vi "Main.vi"(11 "Module Admin":refnum<class "Delacor_lib_QMH_Module Admin.lvclass">) -> ()   [LabVIEW 2020, in "horiba.lvlib" / "DeviceManager.lvlib"]
doc: "This template is based off of the Queued Message Handler design pattern and the Queued Message Handler project template that ships with LabVIEW.\n\nThe main difference is that the queue is private to this module and communication between modules is performed via Broadcast and Request events.\n\nRequest events are wrapped in public API methods and are handled in the Event Handling Loop (EHL) of this VI. Any module can register for Broadcast events sent by this module. The EHL generates messages based on user interface actions.\n\nThe Message Handling Loop (MHL) processes messages generated by the EHL, or by other messages. The messages are string values, so new messages can be added easily to the Message Cases case structure in the MHL. Each message cluster can also provide an optional value for Message Data, which is a variant that can be converted to whatever message-specific data is required.\n_____\nBased on DQMH Project Template 7.0.0.1280."
uses:
  DeviceManager.lvlib
  <vilib>/Delacor/Delacor QMH/Libraries/Message Queue_class/Delacor_lib_QMH_Message Queue.lvclass
  Module Data--cluster.ctl
  <vilib>/Utility/miscctls.llb/LVPointTypeDef.ctl
  <vilib>/Delacor/Delacor QMH/Libraries/Message Queue_class/Delacor_lib_QMH_Enqueue Message (Single).vi
  Stop Argument--cluster.ctl
  <vilib>/Delacor/Delacor QMH/Libraries/Module Admin_class/Delacor_lib_QMH_Module Admin.lvclass
  OpenWebSocketCommunication (Reply Payload)--cluster.ctl
  ICLcommuncationData.ctl
  <vilib>/GPower/Error/GPError.lvlib
  Communicator/Communicator.lvclass
  SendJSONandAskForReply (Reply Payload)--cluster.ctl
  Mono/Monochromator.lvclass
  CCD/CCD.lvclass
  SCD/SCD.lvclass
  DiscoverDevices (Reply Payload)--cluster.ctl
  DevicesList (Reply Payload)--cluster.ctl
  18cac8b0-4f25-4128-b3b0-f125cc614320.vi
  3b3cd88e-03c4-4dd7-b5f0-8a6c9de4e459.vi
  89821459-91c3-422b-9ff8-53e1432d37b0.vi
  <vilib>/Hampel Software Engineering/HSE Logger/hse-logger.lvlib
panel:
  out "error out":errorcluster
  out "Status":string
  in  "Simulate MHL Error":bool
  in  "Simulate EHL Error":bool
  # "Device Manager"
  # "This DQMH module starts the Instrument Control Layer (ICL)\nand proved means to send messages to the ICL via websocket\ncommunication."
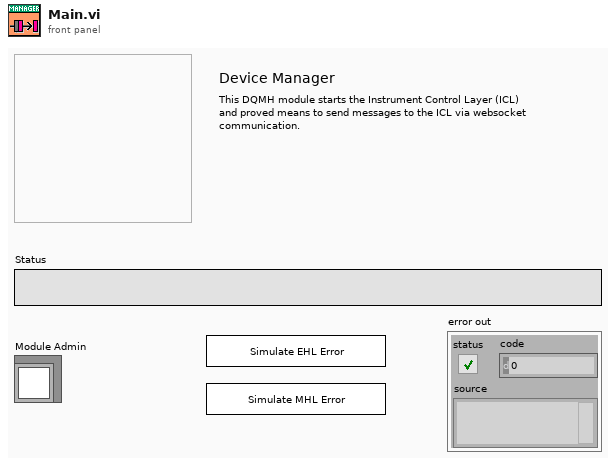
[diagram p1: front panel]
types:
  T1 = typedef "horiba.lvlib/DeviceManager.lvlib/Request Events--cluster.ctl" = cluster{"Stop Module":refnum<user-event>, "Show Panel":refnum<user-event>, "Hide Panel":refnum<user-event>, "Get Module Execution Status":refnum<user-event>, "Show Diagram":refnum<user-event>, "StartICL":refnum<user-event>, "OpenWebSocketCommunication":refnum<user-event>, "Private":cluster{"ICLstartNotification":refnum<user-event>}, "ICLshutdown":refnum<user-event>, "SendJSONandAskForReply":refnum<user-event>, "DiscoverDevices":refnum<user-event>, "DevicesList":refnum<user-event>}
  T2 = typedef "horiba.lvlib/DeviceManager.lvlib/ICLcommuncationData.ctl" = cluster{"Status":string, "ICL.exe started":bool, "Communicator":refnum<class "Communicator.lvclass">}
  T3 = typedef "horiba.lvlib/DeviceManager.lvlib/Module Data--cluster.ctl" = cluster{"Status":string}
  T4 = enum32{"invalid lock state", "Not Locked", "Locked (No Password)", "Password-protected"}
  T5 = typedef "horiba.lvlib/DeviceManager.lvlib/Stop Argument--cluster.ctl" = cluster{"Origin":string, "Exit via Stop Module Req?":bool, "Wait for Module to stop?":bool}
  T6 = typedef "LVPointTypeDef.ctl" = cluster{"Horizontal":i16, "Vertical":i16}
  T7 = enum32{"Invalid", "Standard", "Closed", "Hidden", "Minimized", "Maximized"}
  T8 = typedef "horiba.lvlib/DeviceManager.lvlib/OpenWebSocketCommunication (Reply Payload)--cluster.ctl" = cluster{"Return Headers":variant, "error":errorcluster}
  T9 = typedef "horiba.lvlib/DeviceManager.lvlib/SendJSONandAskForReply (Reply Payload)--cluster.ctl" = cluster{"JSON reply":string, "error":errorcluster}
  T10 = typedef "horiba.lvlib/DeviceManager.lvlib/DiscoverDevices (Reply Payload)--cluster.ctl" = cluster{"Monos":refnum<class "Monochromator.lvclass">[], "CCDs":refnum<class "CCD.lvclass">[], "SCDs":refnum<class "SCD.lvclass">[], "error":errorcluster}
  T11 = typedef "horiba.lvlib/DeviceManager.lvlib/DevicesList (Reply Payload)--cluster.ctl" = cluster{"monochromator results":string, "CCD-results":string, "SCD-results":string, "error":errorcluster}
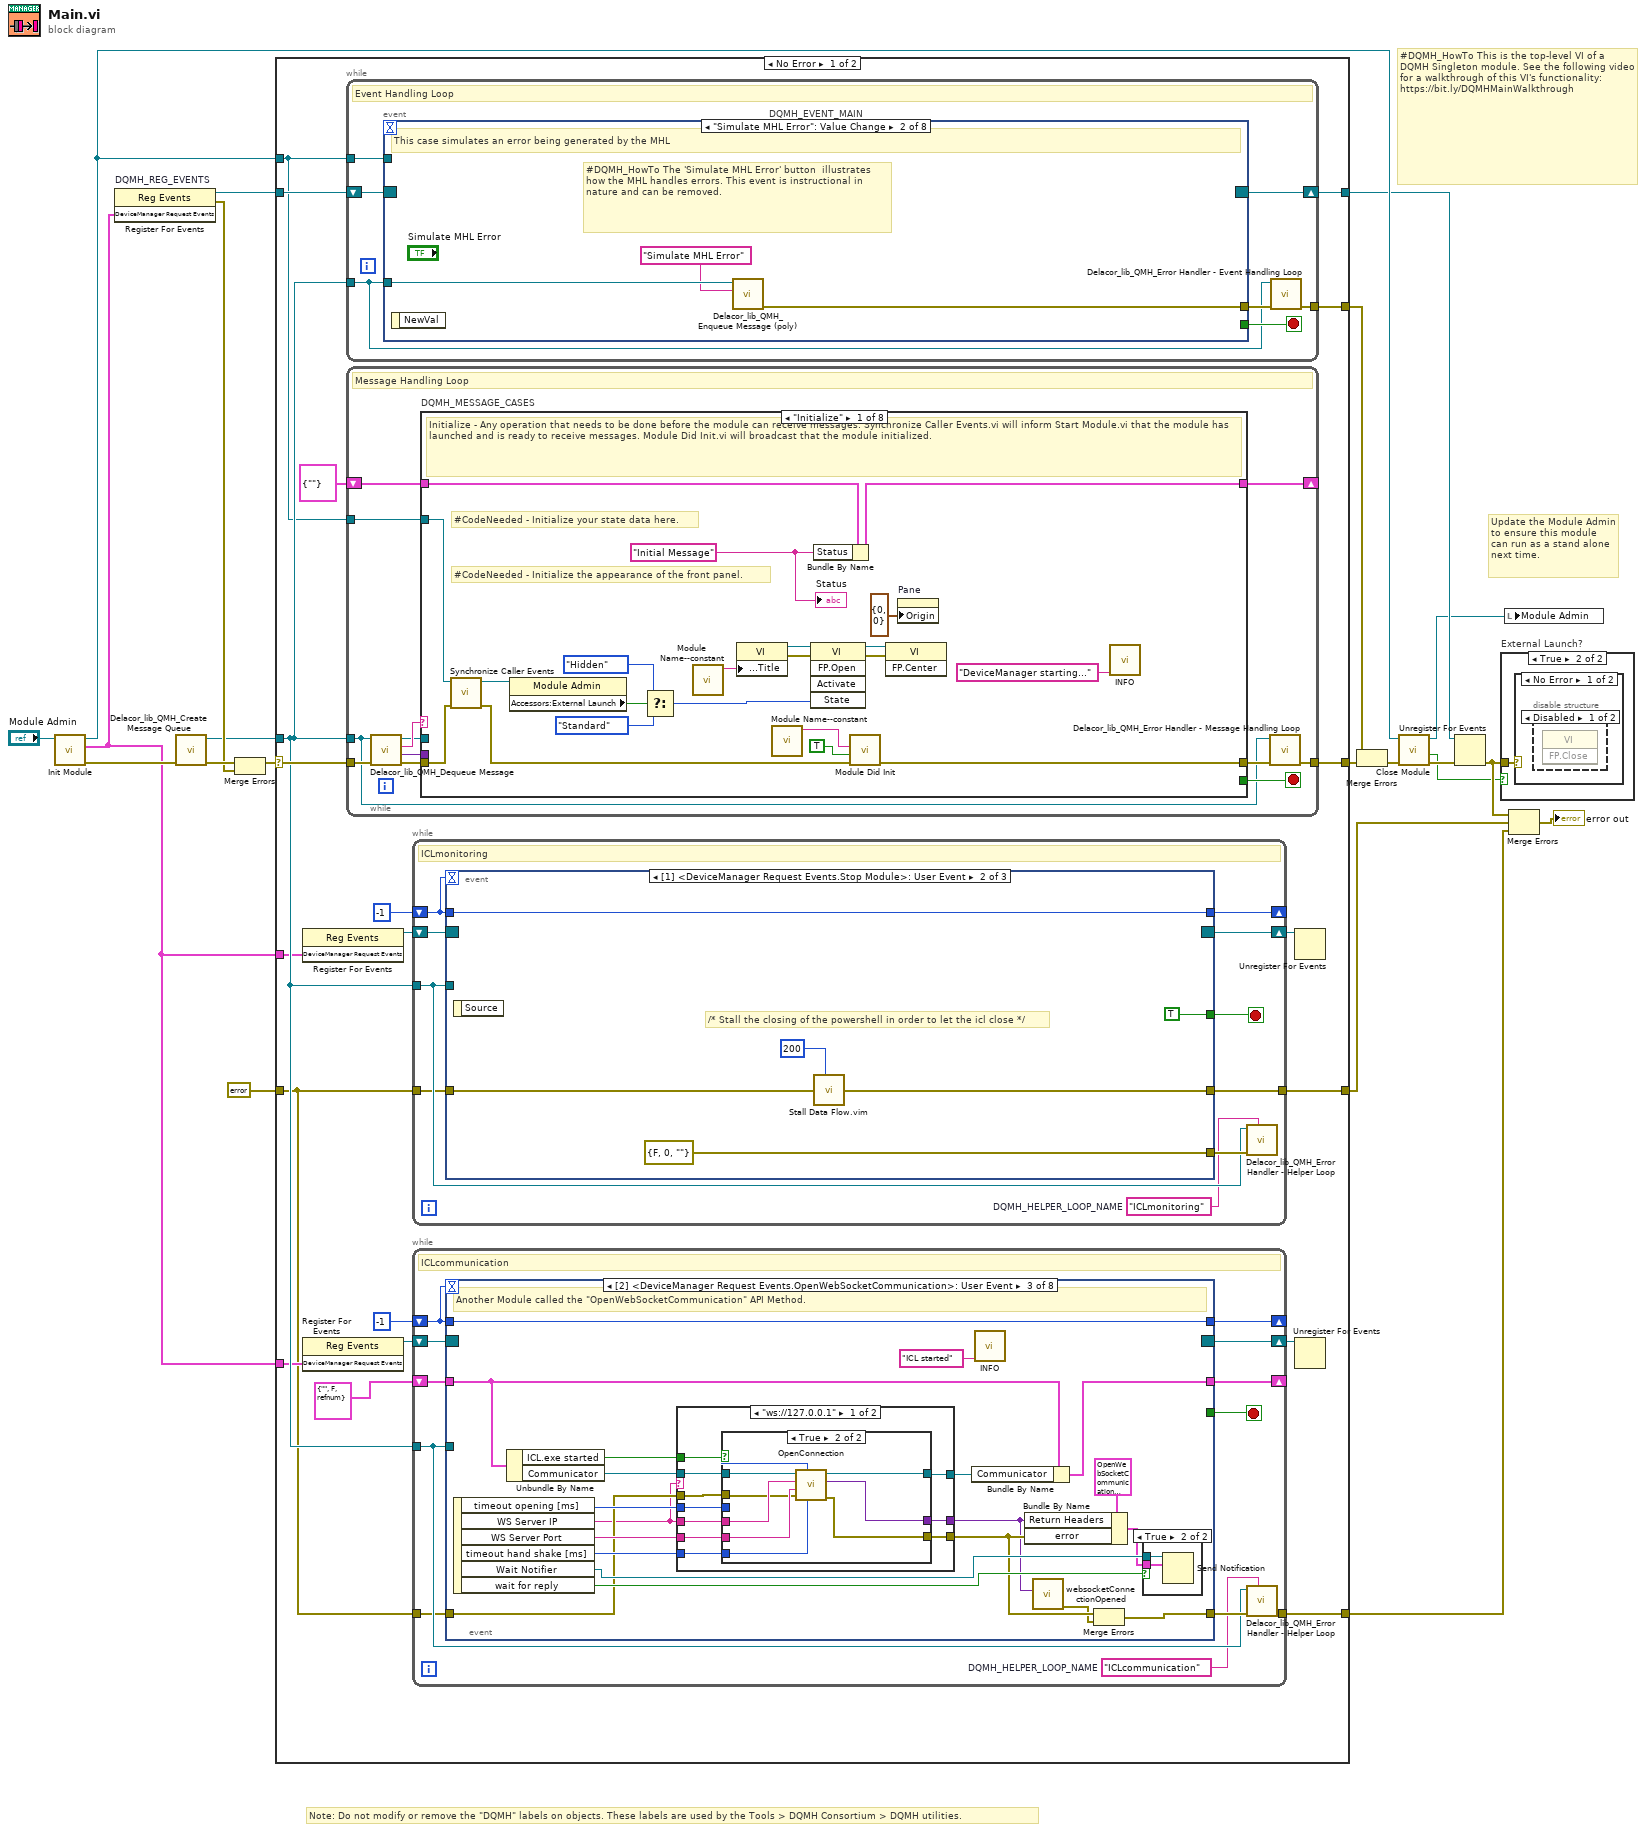
[diagram p0: block diagram]
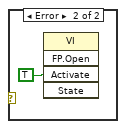
[diagram p4: hidden frame]
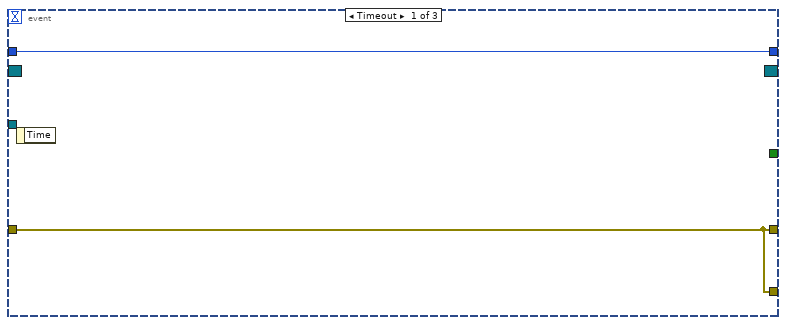
[diagram p5: hidden frame]
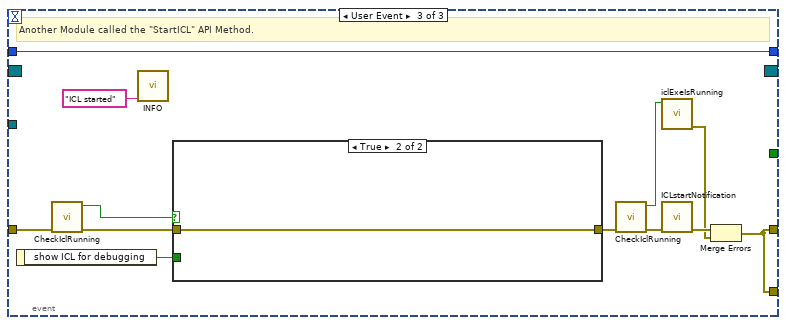
[diagram p6: hidden frame]
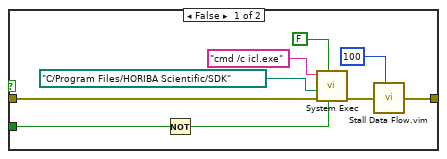
[diagram p7: hidden frame]
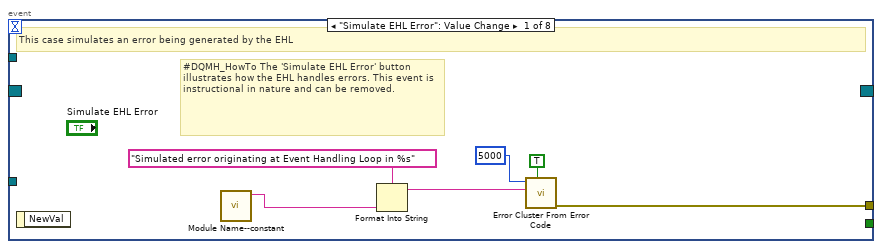
[diagram p8: hidden frame]
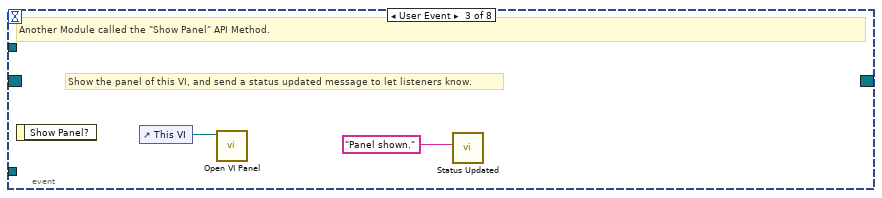
[diagram p9: hidden frame]
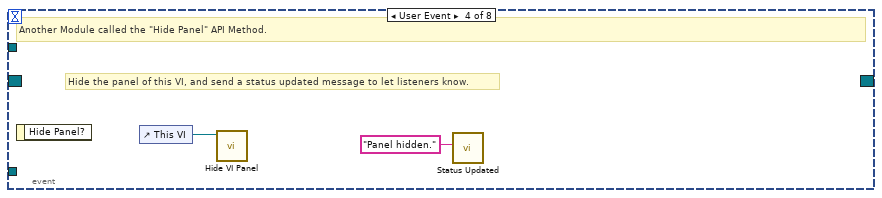
[diagram p10: hidden frame]
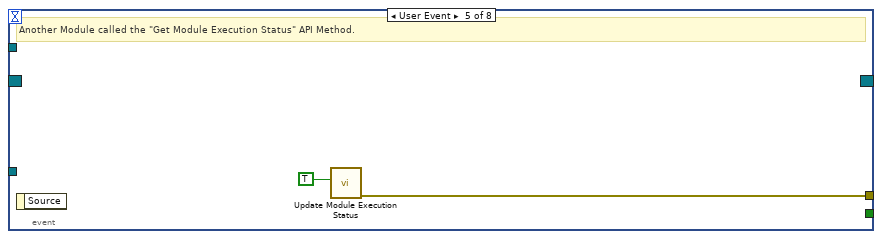
[diagram p11: hidden frame]
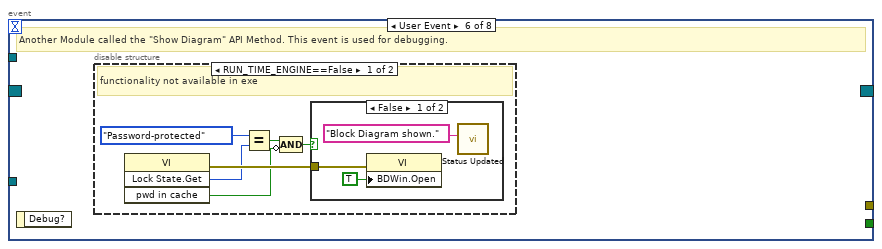
[diagram p12: hidden frame]
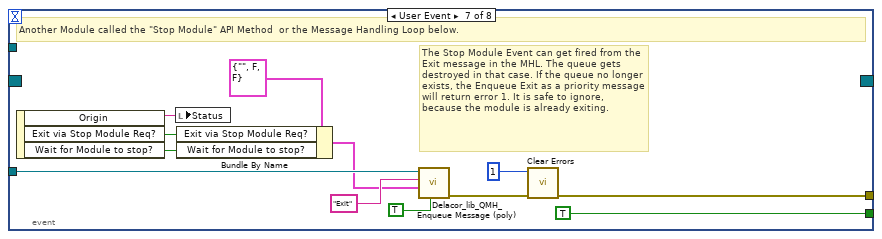
[diagram p15: hidden frame]
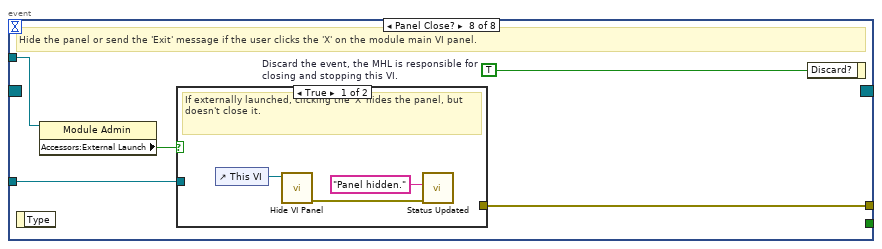
[diagram p16: hidden frame]
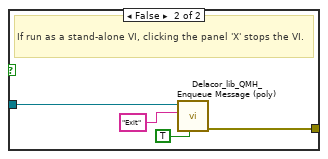
[diagram p17: hidden frame]
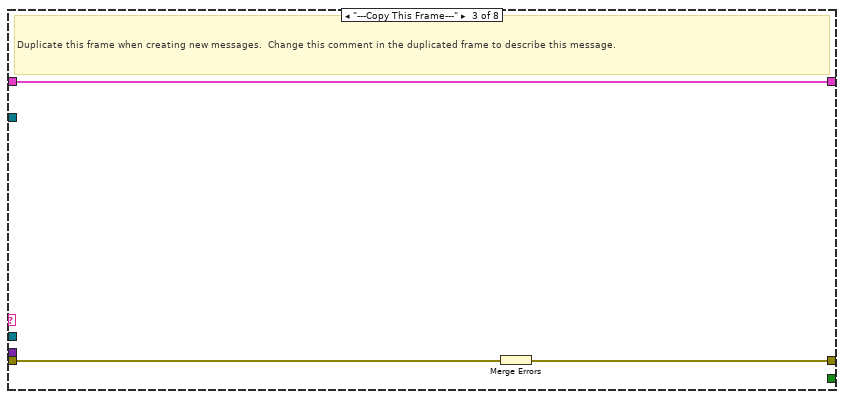
[diagram p19: hidden frame]
diagram:
  # "#DQMH_HowTo This is the top-level VI of a DQMH Singleton module. See the following video for a walkthrough of this VI's functionality: https://bit.ly/DQMHMainWalkthrough"
  # "Note: Do not modify or remove the \"DQMH\" labels on objects. These labels are used by the Tools > DQMH Consortium > DQMH utilities."
  # "Update the Module Admin to ensure this module can run as a stand alone next time."
  n1 = call "Init Module.vi"("Singleton Module Admin in"="Module Admin") -> ("error out"=w20:errorcluster, "DeviceManager Request Events"=w3:T1, "Singleton Module Admin out"=w12:refnum<class "Delacor_lib_QMH_Module Admin.lvclass">)  [unwired: 8 in]
  n2 = register-events "DQMH_REG_EVENTS"(w3) -> (reference out=w10:refnum<event-registration>, error out=w13:errorcluster)  [unwired: 2 in]
  n3 = call <vilib>:"Delacor_lib_QMH_Create Message Queue.vi"("error in"=w20) -> ("error out"=w15:errorcluster, "Message Queue"=w9:refnum<class "Delacor_lib_QMH_Message Queue.lvclass">)  [unwired: 9 in]
  n4 = Merge Errors(w15, w13) -> (w14:errorcluster)
  n5 = case shown="No Error" w14 {
    selector: w14 -> [w39 w402]
    tunnel: [w41 w401] -> w21
    tunnel: [w38 w400] -> w11
    tunnel: w10 -> [w36 w400]
    tunnel: w9 -> [w35 w395]
    tunnel: [w40 _] -> w18
    tunnel: w12 -> [w34 w396]
    tunnel: w3 -> [w33 _]
    tunnel: errorcluster {"status"=FALSE, "code"=0, "source"=""} ("error out") -> [w23 w394]
    tunnel: [w29 w394] -> w5
    tunnel: w3 -> [w28 _]
    tunnel: [w22 _] -> w1
    frame No Error {
      n6 = register-events ("DQMH_HELPER_REGFOREVENTS")(w33) -> (reference out=w31:refnum<event-registration>)  [unwired: 2 in, 1 out]
      n7 = register-events ("DQMH_HELPER_REGFOREVENTS")(w28) -> (reference out=w26:refnum<event-registration>)  [unwired: 2 in, 1 out]
      n8 = while {
        tunnel: w35 -> [w82]
        shift-right: [w85] -> w38
        shift-left: w36 -> [w86]
        tunnel: [w87] -> w40
        tunnel: w34 -> [w83]
        stop <- w84 stop-if-true
        # "Event Handling Loop"
        n9 = event "DQMH_EVENT_MAIN" shown="[1] \"Simulate MHL Error\": Value Change" {
          selector: w86 -> [_ _ _ _ _ _ _ _]
          dyn-events: [_ _ _ _ _ _ _ _] -> w85
          timeout: _ -> [_ _ _ _ _ _ _ _]
          tunnel: [_ _ _ _ _ _ TRUE ("Discard?") _] -> w84
          tunnel: w82 -> [_ w96 _ _ _ _ w120 w127]
          tunnel: [w94 w97 _ _ w103 _ w123 w129] -> w88
          tunnel: w83 -> [_ _ _ _ _ _ _ w126]
          event "Simulate EHL Error": Value Change {
            # "#DQMH_HowTo The 'Simulate EHL Error' button  illustrates how the EHL handles errors. This event is instructional in nature and can be removed."
            # "This case simulates an error being generated by the EHL"
            n10 = event-data() -> ()  [unwired: 1 in, 1 out]
            n11 = call "Module Name--constant.vi"() -> ("Module Name"=w91:string)  [unwired: 11 in]
            n12 = Format Into String(format string="Simulated error originating at Event Handling Loop in %s", w91) -> (resulting string=w92:string)  [unwired: 2 in, 1 out]
            n13 = call <vilib>:"Error Cluster From Error Code.vi"("show call chain? (False)"=TRUE, "error message (\"\")"=w92, "error code (0)"=5000) -> ("error out"=w94:errorcluster)  [unwired: 6 in]
          }
          event "Simulate MHL Error": Value Change {
            # "#DQMH_HowTo The 'Simulate MHL Error' button  illustrates how the MHL handles errors. This event is instructional in nature and can be removed."
            # "This case simulates an error being generated by the MHL"
            n14 = event-data() -> ()  [unwired: 1 in, 1 out]
            n15 = call-poly <vilib>:"Delacor_lib_QMH_Enqueue Message (poly).vi"("Message"="Simulate MHL Error", "Message Queue in"=w96) -> ("error out"=w97:errorcluster)  [unwired: 8 in, 1 out]
          }
          event User Event {
            # "Show the panel of this VI, and send a status updated message to let listeners know."
            # "Another Module called the \"Show Panel\" API Method."
            n16 = event-data() -> ()  [unwired: 1 in, 1 out]
            n17 = control-ref of="This VI"() -> (w99:refnum<vi>)
            n18 = call "Open VI Panel.vi"("VI"=w99) -> ()  [unwired: 10 in, 1 out]
            n19 = call "Status Updated.vi"("Status"="Panel shown." ("format string")) -> ()  [unwired: 10 in, 1 out]
          }
          event User Event {
            # "Hide the panel of this VI, and send a status updated message to let listeners know."
            # "Another Module called the \"Hide Panel\" API Method."
            n20 = event-data() -> ()  [unwired: 1 in, 1 out]
            n21 = control-ref of="This VI"() -> (w101:refnum<vi>)
            n22 = call "Hide VI Panel.vi"("VI"=w101) -> ()  [unwired: 10 in, 1 out]
            n23 = call "Status Updated.vi"("Status"="Panel hidden." ("format string")) -> ()  [unwired: 10 in, 1 out]
          }
          event User Event {
            # "Another Module called the \"Get Module Execution Status\" API Method."
            n24 = event-data() -> ()  [unwired: 1 in, 1 out]
            n25 = call "Update Module Execution Status.vi"("Running?"=TRUE) -> ("error out"=w103:errorcluster)  [unwired: 10 in]
          }
          event User Event {
            # "Another Module called the \"Show Diagram\" API Method. This event is used for debugging."
            n26 = event-data() -> ()  [unwired: 1 in, 1 out]
            n27 = disable-structure shown="RUN_TIME_ENGINE==False" {
              frame condition #0 (active) {
                # "functionality not available in exe"
                n28 = invoke class="VI" method="Lock State.Get"() -> (error out=w109:errorcluster, "Get Lock State"=w108:T4, "pwd in cache"=w105:bool)  [unwired: 4 in, 1 out]
                n29 = Equal?(x=T4."Password-protected", y=w108) -> (x = y?=w106:bool)
                n30 = Compound Arithmetic op=AND(w106, invert w105) -> (w104:bool)
                n31 = case shown="False" w104 {
                  tunnel: w109 -> [w112 _]
                  frame False {
                    n32 = property class="VI"(error in=w112, "BDWin.Open"=TRUE ("Block Diagram Window:Open")) -> ()  [unwired: 1 in, 2 out]
                    n33 = call "Status Updated.vi"("Status"="Block Diagram shown." ("format string")) -> ()  [unwired: 10 in, 1 out]
                  }
                  frame True {
                    # "Password-protected VI, and the password is not in the cache. Do not show the diagram."
                  }
                }
              }
              frame condition #1 {
              }
            }
          }
          event User Event {
            # "The Stop Module Event can get fired from the Exit message in the MHL. The queue gets destroyed in that case. If the queue no longer exists, the Enqueue Exit as a priority message will return error 1. It is safe to ignore, because the module is already exiting."
            # "Another Module called the \"Stop Module\" API Method  or the Message Handling Loop below."
            n34 = event-data() -> ("Origin"=w119:string, "Exit via Stop Module Req?"=w115:bool, "Wait for Module to stop?"=w114:bool)  [unwired: 1 in]
            n35 = local write "Status"(w119) -> ()
            n36 = Bundle By Name(cluster=T5 {"Origin"="", "Exit via Stop Module Req?"=FALSE, "Wait for Module to stop?"=FALSE} ("Stop Argument"), "Exit via Stop Module Req?"=w115, "Wait for Module to stop?"=w114) -> (w113:T5)
            n37 = call-poly <vilib>:"Delacor_lib_QMH_Enqueue Message (poly).vi"("Priority Message? (F)"=TRUE, "Message Data"=w113, "Message"="Exit", "Message Queue in"=w120) -> ("error out"=w124:errorcluster)  [unwired: 6 in, 1 out]
            n38 = call <vilib>:"Clear Errors.vi"("error in (no error)"=w124, "specific error code to clear (0: all)"=1) -> ("error out"=w123:errorcluster)  [unwired: 4 in, 1 out]
          }
          event Panel Close? {
            w128 = TRUE  # Discard the event, the MHL is responsible for closing and stopping this VI.
            # "Hide the panel or send the 'Exit' message if the user clicks the 'X' on the module main VI panel."
            n39 = event-data() -> ()  [unwired: 1 in, 1 out]
            n40 = property class="Module Admin"(reference=w126) -> ("Accessors:External Launch"=w125:bool)  [unwired: 1 in, 2 out]
            n41 = case shown="True" w125 {
              tunnel: w127 -> [_ w135]
              tunnel: [_ w136] -> w129
              frame True {
                # "If externally launched, clicking the 'X' hides the panel, but doesn't close it."
                n42 = control-ref of="This VI"() -> (w132:refnum<vi>)
                n43 = call "Hide VI Panel.vi"("VI"=w132) -> ("error out"=w130:errorcluster)  [unwired: 10 in]
                n44 = call "Status Updated.vi"("error in"=w130, "Status"="Panel hidden." ("format string")) -> ()  [unwired: 9 in, 1 out]
              }
              frame False {
                # "If run as a stand-alone VI, clicking the panel 'X' stops the VI."
                n45 = call-poly <vilib>:"Delacor_lib_QMH_Enqueue Message (poly).vi"("Priority Message? (F)"=TRUE, "Message"="Exit", "Message Queue in"=w135) -> ("error out"=w136:errorcluster)  [unwired: 7 in, 1 out]
              }
            }
            n46 = event-data("Discard?"=w128) -> ()  [unwired: 1 in, 1 out]
          }
        }
        n47 = call-dynamic "Delacor_lib_QMH_Error Handler - Event Handling Loop.vi"("error in"=w88, "Message Queue in"=w82) -> ("dup error in"=w87:errorcluster)  [unwired: 8 in, 1 out]
      }
      n48 = while {
        tunnel: w35 -> [w137]
        shift-right: [w143] -> _
        shift-left: T3 {"Status"=""} ("Data Cluster") -> [w144]
        tunnel: w39 -> [w147]
        tunnel: [w145] -> w41
        tunnel: w34 -> [w138]
        stop <- w142 stop-if-true
        # "Message Handling Loop"
        n49 = call-dynamic "Delacor_lib_QMH_Dequeue Message.vi"("error in"=w147, "Message Queue in"=w137) -> ("error out"=w146:errorcluster, "Message Data"=w140:variant, "Message"=w141:string, "Message Queue out"=w139:refnum<class "Delacor_lib_QMH_Message Queue.lvclass">)  [unwired: 6 in]
        n50 = case "DQMH_MESSAGE_CASES" shown="\"Initialize\"" w141 {
          selector: w141 -> [_ _ _ _ _ _ _ w224]
          tunnel: w139 -> [_ _ _ _ _ w190 w212 _]
          tunnel: w146 -> [w167 w171 w174 w176 w185 w197 w218 w227]
          tunnel: [w165 w171 w173 w176 w184 w193 w213 w228] -> w148
          tunnel: w144 -> [w156 w170 w172 w175 w182 w192 w211 w225]
          tunnel: [w155 w170 w172 w175 w182 w192 w211 w225] -> w143
          tunnel: [_ _ _ _ _ _ w210 _] -> w142
          tunnel: w140 -> [_ _ _ _ _ w191 w209 _]
          tunnel: w138 -> [w157 _ _ _ _ w189 w204 _]
          frame "Initialize" {
            w151 = "Initial Message" ("Initial Message")
            # "#CodeNeeded - Initialize the appearance of the front panel."
            # "#CodeNeeded - Initialize your state data here."
            # "Initialize - Any operation that needs to be done before the module can receive messages. Synchronize Caller Events.vi will inform Start Module.vi that the module has launched and is ready to receive messages. Module Did Init.vi will broadcast that the module initialized."
            n51 = call "Synchronize Caller Events.vi"("error in"=w167, "Singleton Module Admin in"=w157) -> ("error out"=w166:errorcluster, "Singleton Module Admin out"=w152:refnum<class "Delacor_lib_QMH_Module Admin.lvclass">)  [unwired: 8 in]
            n52 = property class="Module Admin"(reference=w152) -> ("Accessors:External Launch"=w161:bool)  [unwired: 1 in, 2 out]
            n53 = Select(t=T7."Hidden" ("State"), s=w161, f=T7."Standard" ("State")) -> (s? t:f=w158:T7)
            n54 = call "Module Name--constant.vi"() -> ("Module Name"=w164:string)  [unwired: 11 in]
            n55 = property class="VI"("Front Panel.Title"=w164) -> (reference out=w163:refnum<vi>, error out=w169:errorcluster)  [unwired: 2 in]
            n56 = call "Module Name--constant.vi"() -> ("Module Name"=w153:string)  [unwired: 11 in]
            n57 = invoke class="VI" method="FP.Open"(reference=w163, error in=w169, "State"=w158) -> (reference out=w162:refnum<vi>, error out=w168:errorcluster)  [unwired: 2 in, 3 out]
            n58 = Bundle By Name(cluster=w156, "Status"=w151) -> (w155:T3)
            n59 = call "Module Did Init.vi"("error in"=w166, "Initialized?"=TRUE, "Origin"=w153) -> ("error out"=w165:errorcluster)  [unwired: 8 in]
            n60 = invoke class="VI" method="FP.Center"(reference=w162, error in=w168) -> ()  [unwired: 1 in, 3 out]
            n61 = property on="Pane" class="Pane"("Origin"=T6 {"Horizontal"=0, "Vertical"=0}) -> ()  [unwired: 2 in, 2 out]
            n62 = call <vilib>:"INFO.vi"("Message"="DeviceManager starting...") -> ()  [unwired: 10 in, 1 out]
            "Status" <- w151
          }
          frame "---Module Specific---" {
            # "Separator -- The following cases handle messages specific to this Module."
          }
          frame "---Copy This Frame---" {
            # "Duplicate this frame when creating new messages.  Change this comment in the duplicated frame to describe this message."
            n63 = Merge Errors(w174) -> (w173:errorcluster)
          }
          frame "---Exit and Error Handling---" {
            # "Separator - The following cases handle errors and exit messages."
          }
          frame "Simulate MHL Error" {
            # "#DQMH_HowTo The 'Simulate MHL Error' button  illustrates how the MHL handles errors. This event is instructional in nature and can be removed."
            # "Simulate an error occurring at the MHL"
            n64 = call "Module Name--constant.vi"() -> ("Module Name"=w178:string)  [unwired: 11 in]
            n65 = Format Into String(format string="Simulated error originating at Message Handling Loop in %s", w178) -> (resulting string=w179:string)  [unwired: 2 in, 1 out]
            n66 = call <vilib>:"Error Cluster From Error Code.vi"("show call chain? (False)"=TRUE, "error message (\"\")"=w179, "error code (0)"=5001) -> ("error out"=w183:errorcluster)  [unwired: 6 in]
            n67 = Merge Errors(w185, w183) -> (w184:errorcluster)
          }
          frame "Error" {
            # "#CodeRecommended - If the module is running in standalone mode (External Launch = FALSE), this code will pop up an error dialog and call the 'Exit' message if an error occurs. Add more fine-grained error management here."
            # "Error - Check the error message data and respond accordingly. This message is sent by the \"Error Handler\" VIs at the end of each loop in this application."
            n68 = property class="Module Admin"(reference=w189) -> ("Accessors:External Launch"=w188:bool)  [unwired: 1 in, 2 out]
            n69 = Variant To Data(error in=w197, type=errorcluster {"status"=FALSE, "code"=0, "source"=""} ("error constant"), Variant=w191) -> (data=w187:errorcluster, error out=w195:errorcluster)
            n70 = local write "error out"(w187) -> ()
            n71 = call <vilib>:"ERROR.vi"("Message"="DeviceHandler Error", "error in"=w187) -> ()  [unwired: 9 in, 1 out]
            n72 = call "Error Reported.vi"("Error"=w187) -> ()  [unwired: 10 in, 1 out]
            n73 = case shown="True" w188 {
              tunnel: [w202 _] -> w194
              tunnel: w190 -> [w200 _]
              tunnel: w187 -> [w201 _]
              frame False {
                n74 = disable-structure shown="Default" {
                  disable-tunnel: w201 -> [w203 _]
                  frame condition #0 (active) {
                    # "If the module is running standalone, then pop up an error dialog and call the \"Exit\" message."
                    n75 = call <vilib>:"Simple Error Handler.vi"("error in (no error)"=w203) -> ()  [unwired: 4 in, 5 out]
                  }
                  frame condition #1 {
                    # "To prevent the Simple Error Handler VI from being loaded (e.g. when deploying to a Real-Time target), add the Conditional Disable Symbol \"DQMH_Disable_SEH\" to your project and set it to TRUE."
                  }
                }
                n76 = call-poly <vilib>:"Delacor_lib_QMH_Enqueue Message (poly).vi"("Priority Message? (F)"=TRUE, "Message"="Exit", "Message Queue in"=w200) -> ("error out"=w202:errorcluster)  [unwired: 7 in, 1 out]
              }
              frame True {
                # "If the module was launched externally, calling the Error Reported broadcast VI is the only action performed by the \"Error\" message. The module's caller can then process the error appropriately."
              }
            }
            n77 = Merge Errors(w195, w194) -> (w193:errorcluster)
          }
          frame "Exit" {
            w208 = 91  # 91: not all Exit messages will have an argument
            w210 = TRUE  # Stop the VI
            # "Release the message queue reference"
            # "#CodeNeeded - Add any required cleanup code here."
            # "Exit - Exit the application."
            n78 = Variant To Data(error in=w218, type=T5 {"Origin"="", "Exit via Stop Module Req?"=FALSE, "Wait for Module to stop?"=FALSE} ("Stop Argument"), Variant=w209) -> (data=w206:T5, error out=w215:errorcluster)
            n79 = call <vilib>:"Clear Errors.vi"("error in (no error)"=w215, "specific error code to clear (0: all)"=w208) -> ("error out"=w217:errorcluster)  [unwired: 4 in, 1 out]
            n80 = control-ref of="This VI"() -> (w205:refnum<vi>)
            n81 = call-dynamic "Delacor_lib_QMH_Release Message Queue.vi"("error in"=w217, "Message Queue"=w212) -> ("error out"=w216:errorcluster)  [unwired: 9 in]
            n82 = call "Handle Exit.vi"("Stop Argument"=w206, "Admin in"=w204, "VI reference"=w205) -> ("error out"=w214:errorcluster)  [unwired: 7 in, 1 out]
            n83 = Merge Errors(w216, w214) -> (w213:errorcluster)
            n84 = call "Error Reported.vi"("Error"=w213) -> ()  [unwired: 10 in, 1 out]
          }
          frame Default {
            # "'Default' case only runs if there is a message that isn't defined in any of the other cases.  Output a programming error."
            n85 = call "Module Name--constant.vi"() -> ("Module Name"=w223:string)  [unwired: 11 in]
            n86 = Format Into String(format string="The invalid message string \"%s\" was received in the Message Handling Loop for module \"%s\".", w224, w223) -> (resulting string=w219:string)  [unwired: 2 in, 1 out]
            n87 = call <vilib>:"Error Cluster From Error Code.vi"("show call chain? (False)"=TRUE, "error message (\"\")"=w219, "error code (0)"=1) -> ("error out"=w226:errorcluster)  [unwired: 6 in]
            n88 = Merge Errors(w227, w226) -> (w228:errorcluster)
          }
        }
        n89 = call-dynamic "Delacor_lib_QMH_Error Handler - Message Handling Loop.vi"("error in"=w148, "Message Queue in"=w137) -> ("dup error in"=w145:errorcluster)  [unwired: 8 in, 1 out]
      }
      n90 = while "DQMH_HELPER_LOOP" {
        shift-right: [w51] -> _
        shift-left: -1 -> [w50]
        shift-right: [w48] -> w32
        shift-left: w31 -> [w49]
        tunnel: w35 -> [w45]
        tunnel: w23 -> [w43]
        tunnel: [w42] -> w29
        stop <- w47 stop-if-true
        w44 = "ICLmonitoring"  # DQMH_HELPER_LOOP_NAME
        # "ICLmonitoring"
        n91 = event "DQMH_HELPER_EVENT_STRUCTURE" shown="[1] <DeviceManager Request Events.Stop Module>: User Event" {
          selector: w49 -> [_ _ _]
          dyn-events: [_ _ _] -> w48
          timeout: w50 -> [_ _ _]
          tunnel: w50 -> [w53 w59 w71]
          tunnel: [w53 w59 w71] -> w51
          tunnel: [_ TRUE _] -> w47
          tunnel: [w52 errorcluster {"status"=FALSE, "code"=0, "source"=""} ("error constant") w65] -> w46
          tunnel: w45 -> [_ _ _]
          tunnel: w43 -> [w52 w56 w69]
          tunnel: [w52 w55 w65] -> w42
          event Timeout {
            n92 = event-data() -> ()  [unwired: 1 in, 1 out]
          }
          event User Event {
            # "/* Stall the closing of the powershell in order to let the icl close */"
            n93 = event-data() -> ()  [unwired: 1 in, 1 out]
            n94 = call "Stall Data Flow.vim"("value in"=w56, "milliseconds to wait"=u32 200) -> ("value out"=w55:errorcluster)  [unwired: 1 out]
          }
          event User Event {
            # "Another Module called the \"StartICL\" API Method."
            n95 = event-data() -> ("show ICL for debugging"=w67:bool)  [unwired: 1 in]
            n96 = call "CheckIclRunning.vi"("error in (no error)"=w69) -> ("error out"=w68:errorcluster, "icl.exe running"=w66:bool)  [unwired: 9 in]
            n97 = call <vilib>:"INFO.vi"("Message"="ICL started") -> ()  [unwired: 10 in, 1 out]
            n98 = case shown="True" w66 {
              tunnel: [w73 w81] -> w63
              tunnel: w68 -> [w77 w81]
              tunnel: w67 -> [w75 _]
              frame False {
                n99 = Not(x=w75) -> (.not. x?=w74:bool)
                n100 = call <vilib>:"System Exec.vi"("run minimized? (F)"=w74, "wait until completion? (T)"=FALSE, "error in (no error)"=w77, "working directory"=path "C:/Program Files/HORIBA Scientific/SDK", "command line"="cmd /c icl.exe") -> ("error out"=w76:errorcluster)  [unwired: 3 in, 3 out]
                n101 = call "Stall Data Flow.vim"("value in"=w76, "milliseconds to wait"=u32 100) -> ("value out"=w73:errorcluster)  [unwired: 1 out]
              }
              frame True {
              }
            }
            n102 = call "CheckIclRunning.vi"("error in (no error)"=w63) -> ("error out"=w62:errorcluster, "icl.exe running"=w61:bool)  [unwired: 9 in]
            n103 = call "iclExeIsRunning.vi"("iclWasAlreadyRunning"=w61) -> ("error out"=w64:errorcluster)  [unwired: 10 in]
            n104 = call "ICLstartNotification.vi"("error in"=w62) -> ("error out"=w70:errorcluster)  [unwired: 10 in]
            n105 = Merge Errors(w70, w64) -> (w65:errorcluster)
          }
        }
        n106 = call-dynamic "Delacor_lib_QMH_Error Handler - Helper Loop.vi"("Error Debug"=w44, "error in"=w46, "Message Queue in"=w45) -> ()  [unwired: 7 in, 2 out]
      }
      n107 = while "DQMH_HELPER_LOOP" {
        shift-right: [w240] -> _
        shift-left: -1 -> [w239]
        shift-right: [w237] -> w27
        shift-left: w26 -> [w238]
        tunnel: w35 -> [w234]
        shift-right: [w231] -> _
        shift-left: T2 {"Status"="", "ICL.exe started"=FALSE, "Communicator"=refnum} ("Data Cluster") -> [w232]
        tunnel: [w230] -> w22
        tunnel: w23 -> [w229]
        stop <- w236 stop-if-true
        w233 = "ICLcommunication"  # DQMH_HELPER_LOOP_NAME
        # "ICLcommunication"
        n108 = event "DQMH_HELPER_EVENT_STRUCTURE" shown="[2] <DeviceManager Request Events.OpenWebSocketCommunication>: User Event" {
          selector: w238 -> [_ _ _ _ _ _ _ _]
          dyn-events: [_ _ _ _ _ _ _ _] -> w237
          timeout: w239 -> [_ _ _ _ _ _ _ _]
          tunnel: w239 -> [w242 w248 w274 w313 w329 w344 w371 w391]
          tunnel: [w242 w248 w274 w313 w329 w344 w371 w391] -> w240
          tunnel: [_ TRUE _ _ _ _ _ _] -> w236
          tunnel: [_ errorcluster {"status"=FALSE, "code"=0, "source"=""} ("error constant") w258 _ w314 w334 w349 w375] -> w235
          tunnel: w234 -> [_ _ _ _ _ _ _ _]
          tunnel: w232 -> [w241 w244 w263 w312 w322 w339 w356 w376]
          tunnel: [w241 w244 w264 w311 w323 w333 w355 w376] -> w231
          tunnel: w229 -> [_ _ w260 _ w326 w336 w359 w385]
          event Timeout {
            n109 = event-data() -> ()  [unwired: 1 in, 1 out]
          }
          event User Event {
            n110 = event-data() -> ()  [unwired: 1 in, 1 out]
            n111 = Unbundle By Name(w244) -> ("ICL.exe started"=w243:bool, "Communicator"=w245:refnum<class "Communicator.lvclass">)
            n112 = case shown="True" w243 {
              tunnel: w245 -> [_ w254]
              frame False {
              }
              frame True {
                n113 = call-dynamic "SendAndAskForReply.vi"("String to be sent"="{\"id\":9999, \"command\":\"icl_shutdown\"}", "Communicator in"=w254) -> ("error out"=w251:errorcluster, "Communicator out"=w252:refnum<class "Communicator.lvclass">)  [unwired: 7 in, 1 out]
                n114 = call-dynamic "CloseConnection.vi"("error in (no error)"=w251, "Communicator in"=w252) -> ("error out"=w250:errorcluster)  [unwired: 8 in, 1 out]
                n115 = call <vilib>:"INFO.vi"("Message"="ICL communication stopped") -> ()  [unwired: 10 in, 1 out]
                n116 = call <vilib>:"Clear Errors.vi"("error in (no error)"=w250) -> ()  [unwired: 5 in, 2 out]
              }
            }
          }
          event User Event {
            # "Another Module called the \"OpenWebSocketCommunication\" API Method."
            n117 = event-data() -> ("timeout opening [ms]"=w265:i32, "WS Server IP"=w256:string, "WS Server Port"=w267:string, "timeout hand shake [ms]"=w266:i32, "Wait Notifier"=w273:refnum<notifier>, "wait for reply"=w272:bool)  [unwired: 1 in]
            n118 = Unbundle By Name(w263) -> ("ICL.exe started"=w269:bool, "Communicator"=w268:refnum<class "Communicator.lvclass">)
            n119 = case shown="\"ws://127.0.0.1\"" w256 {
              tunnel: w269 -> [w284 _]
              tunnel: w268 -> [w283 w307]
              tunnel: w267 -> [w282 w306]
              tunnel: w256 -> [w281 w305]
              tunnel: w266 -> [w280 w304]
              tunnel: w265 -> [w279 w303]
              tunnel: [w278 w302] -> w262
              tunnel: [w277 w301] -> w261
              tunnel: w260 -> [w276 w300]
              tunnel: [w275 w299] -> w259
              frame "ws://127.0.0.1" {
                n120 = case shown="True" w284 {
                  tunnel: [w287 w293] -> w277
                  tunnel: [variant ("Return Headers") w292] -> w275
                  tunnel: w283 -> [w285 w298]
                  tunnel: w282 -> [_ w297]
                  tunnel: w281 -> [_ w296]
                  tunnel: w280 -> [_ w295]
                  tunnel: w279 -> [_ w294]
                  tunnel: [w285 w291] -> w278
                  tunnel: w276 -> [_ w290]
                  frame False {
                    n121 = call <vilib>:"SetError.vi"("Error description"="ICL.exe not running,\ncall ICL Start before establishing the communication", "Error code"=5301) -> ("Error out"=w287:errorcluster)  [unwired: 9 in]
                  }
                  frame True {
                    n122 = call-dynamic "OpenConnection.vi"("timeout hand shake [ms]"=w295, "timeout opening [ms]"=w294, "error in (no error)"=w290, "WS Server Port"=w297, "WS Server IP"=w296, "Communicator in"=w298) -> ("error out"=w293:errorcluster, "Return Headers"=w292:variant, "Communicator out"=w291:refnum<class "Communicator.lvclass">)  [unwired: 3 in]
                  }
                }
              }
              frame Default {
                n123 = call-dynamic "OpenConnection.vi"("timeout hand shake [ms]"=w304, "timeout opening [ms]"=w303, "error in (no error)"=w300, "WS Server Port"=w306, "WS Server IP"=w305, "Communicator in"=w307) -> ("error out"=w301:errorcluster, "Return Headers"=w299:variant, "Communicator out"=w302:refnum<class "Communicator.lvclass">)  [unwired: 3 in]
              }
            }
            n124 = Bundle By Name(cluster=w263, "Communicator"=w262) -> (w264:T2)
            n125 = call <vilib>:"INFO.vi"("Message"="ICL started") -> ()  [unwired: 10 in, 1 out]
            n126 = Bundle By Name(cluster=T8 {"Return Headers"=variant, "error"={"status"=FALSE, "code"=0, "source"=""}} ("OpenWebSocketCommunication (Reply Payload)"), "Return Headers"=w259, "error"=w261) -> (w271:T8)
            n127 = call "websocketConnectionOpened.vi"("Return Headers"=w259) -> ("error out"=w257:errorcluster)  [unwired: 10 in]
            n128 = Merge Errors(w261, w257) -> (w258:errorcluster)
            n129 = case "DQMH_FIRE_NOTIFIER" shown="True" w272 {
              tunnel: w273 -> [_ w309]
              tunnel: w271 -> [_ w308]
              frame False {
              }
              frame True {
                n130 = Send Notification(notification=w308, notifier=w309) -> ()  [unwired: 1 in, 2 out]
              }
            }
          }
          event User Event {
            # "This module called the \"Private.ICLstartNotification\" private request."
            n131 = event-data() -> ()  [unwired: 1 in, 1 out]
            n132 = Bundle By Name(cluster=w312, "ICL.exe started"=TRUE) -> (w311:T2)
          }
          event User Event {
            # "Another Module called the \"ICLshutdown\" API Method."
            n133 = event-data() -> ()  [unwired: 1 in, 1 out]
            n134 = Unbundle By Name(w322) -> ("Communicator"=w328:refnum<class "Communicator.lvclass">)
            n135 = call-dynamic "SendAndAskForReply.vi"("error in (no error)"=w326, "String to be sent"="{\"id\":9999, \"command\":\"icl_shutdown\"}", "Communicator in"=w328) -> ("error out"=w319:errorcluster, "Communicator out"=w325:refnum<class "Communicator.lvclass">)  [unwired: 6 in, 1 out]
            n136 = call-dynamic "CloseConnection.vi"("Communicator in"=w325) -> ("error out"=w324:errorcluster)  [unwired: 9 in, 1 out]
            n137 = call <vilib>:"Clear Errors.vi"("error in (no error)"=w324) -> ()  [unwired: 5 in, 2 out]
            n138 = Bundle By Name(cluster=w322, "ICL.exe started"=FALSE, "Communicator"=refnum<class "Communicator.lvclass"> refnum) -> (w323:T2)
            n139 = call "Stall Data Flow.vim"("value in"=w319, "milliseconds to wait"=u32 500) -> ("value out"=w317:errorcluster)  [unwired: 1 out]
            n140 = call "CheckIclRunning.vi"("error in (no error)"=w317) -> ("error out"=w315:errorcluster, "icl.exe running"=w316:bool)  [unwired: 9 in]
            n141 = call "iclExeIsRunning.vi"("error in"=w315, "iclWasAlreadyRunning"=w316) -> ("error out"=w314:errorcluster)  [unwired: 9 in]
          }
          event User Event {
            # "Another Module called the \"SendJSONandAskForReply\" API Method."
            n142 = event-data() -> ("JSON to be sent"=w337:string, "Delay between send and receive [ms]"=w331:i32, "Wait Notifier"=w343:refnum<notifier>, "wait for reply"=w342:bool)  [unwired: 1 in]
            n143 = Unbundle By Name(w339) -> ("Communicator"=w338:refnum<class "Communicator.lvclass">)
            n144 = call-dynamic "SendAndAskForReply.vi"("Delay between send and receive [ms]"=w331, "error in (no error)"=w336, "timeout for receiving data [ms]"=300, "String to be sent"=w337, "Communicator in"=w338) -> ("error out"=w334:errorcluster, "Data"=w335:string, "Communicator out"=w332:refnum<class "Communicator.lvclass">)  [unwired: 4 in]
            n145 = Bundle By Name(cluster=w339, "Communicator"=w332) -> (w333:T2)
            n146 = Bundle By Name(cluster=T9 {"JSON reply"="", "error"={"status"=FALSE, "code"=0, "source"=""}} ("SendJSONandAskForReply (Reply Payload)"), "JSON reply"=w335, "error"=w334) -> (w341:T9)
            n147 = case "DQMH_FIRE_NOTIFIER" shown="True" w342 {
              tunnel: w343 -> [_ w346]
              tunnel: w341 -> [_ w345]
              frame False {
              }
              frame True {
                n148 = Send Notification(notification=w345, notifier=w346) -> ()  [unwired: 1 in, 2 out]
              }
            }
          }
          event User Event {
            # "Another Module called the \"DiscoverDevices\" API Method."
            n149 = event-data() -> ("Wait Notifier"=w370:refnum<notifier>, "wait for reply"=w369:bool, "timeout for discovering devices [ms]"=w353:i32)  [unwired: 1 in]
            n150 = Unbundle By Name(w356) -> ("Communicator"=w362:refnum<class "Communicator.lvclass">)
            n151 = call "AskForConnectedMonos.vi"("DiscoverDevices in"=T10 {"Monos"=[], "CCDs"=[], "SCDs"=[], "error"={"status"=FALSE, "code"=0, "source"=""}}, "error in (no error)"=w359, "timeout for receiving data [ms]"=w353, "Communicator in"=w362) -> ("error out"=w358:errorcluster, "Monos"=w352:refnum<class "Monochromator.lvclass">[], "DiscoverDevices out"=w360:T10, "Communicator out"=w361:refnum<class "Communicator.lvclass">)  [unwired: 4 in]
            n152 = call "AskForConnectedCCDs.vi"("DiscoverDevices in"=w360, "error in (no error)"=w358, "timeout for receiving data [ms]"=w353, "Communicator in"=w361) -> ("error out"=w366:errorcluster, "CCDs"=w351:refnum<class "CCD.lvclass">[], "DiscoverDevices out"=w367:T10, "Communicator out"=w368:refnum<class "Communicator.lvclass">)  [unwired: 4 in]
            n153 = call "AskForConnectedSCDs.vi"("DiscoverDevices in"=w367, "error in (no error)"=w366, "timeout for receiving data [ms]"=w353, "Communicator in"=w368) -> ("error out"=w365:errorcluster, "SCDs"=w350:refnum<class "SCD.lvclass">[], "DiscoverDevices out"=w364:T10, "Communicator out"=w354:refnum<class "Communicator.lvclass">)  [unwired: 4 in]
            n154 = Bundle By Name(cluster=w364, "error"=w365) -> (w357:T10)
            n155 = Bundle By Name(cluster=w356, "Communicator"=w354) -> (w355:T2)
            n156 = case "DQMH_FIRE_NOTIFIER" shown="True" w369 {
              tunnel: w370 -> [_ w374]
              tunnel: w357 -> [_ w373]
              tunnel: [_ w372] -> w347
              frame False {
              }
              frame True {
                n157 = Send Notification(notification=w373, notifier=w374) -> (error out=w372:errorcluster)  [unwired: 1 in, 1 out]
              }
            }
            n158 = call "devicesDiscovered.vi"("SCDs"=w350, "CCDs"=w351, "Monos"=w352) -> ("error out"=w348:errorcluster)  [unwired: 8 in]
            n159 = Merge Errors(w359, w348, w347) -> (w349:errorcluster)
          }
          event User Event {
            # "Another Module called the \"DevicesList\" API Method."
            n160 = event-data() -> ("Time out [ms]"=w377:i32, "Wait Notifier"=w390:refnum<notifier>, "wait for reply"=w389:bool)  [unwired: 1 in]
            n161 = Unbundle By Name(w376) -> ("Communicator"=w386:refnum<class "Communicator.lvclass">)
            n162 = call "MonoList.vi"("error in (no error)"=w385, "Delay between send and receive [ms]"=w377, "Communicator in"=w386) -> ("error out"=w382:errorcluster, "results-JSON"=w378:string, "Communicator out"=w384:refnum<class "Communicator.lvclass">)  [unwired: 5 in, 1 out]
            n163 = call "CCDList.vi"("error in (no error)"=w382, "Delay between send and receive [ms]"=w377, "Communicator in"=w384) -> ("error out"=w381:errorcluster, "results-JSON"=w380:string, "Communicator out"=w383:refnum<class "Communicator.lvclass">)  [unwired: 5 in, 1 out]
            n164 = call "SCDList.vi"("error in (no error)"=w381, "Delay between send and receive [ms]"=w377, "Communicator in"=w383) -> ("error out"=w375:errorcluster, "results-JSON"=w379:string)  [unwired: 5 in, 2 out]
            n165 = Bundle By Name(cluster=T11 {"monochromator results"="", "CCD-results"="", "SCD-results"="", "error"={"status"=FALSE, "code"=0, "source"=""}} ("DevicesList (Reply Payload)"), "SCD-results"=w379, "CCD-results"=w380, "monochromator results"=w378, "error"=w375) -> (w388:T11)
            n166 = case "DQMH_FIRE_NOTIFIER" shown="True" w389 {
              tunnel: w390 -> [_ w393]
              tunnel: w388 -> [_ w392]
              frame False {
              }
              frame True {
                n167 = Send Notification(notification=w392, notifier=w393) -> ()  [unwired: 1 in, 2 out]
              }
            }
          }
        }
        n168 = call-dynamic "Delacor_lib_QMH_Error Handler - Helper Loop.vi"("Error Debug"=w233, "error in"=w235, "Message Queue in"=w234) -> ("dup error in"=w230:errorcluster)  [unwired: 7 in, 1 out]
      }
      n169 = Unregister For Events(event registration refnum=w32) -> ()  [unwired: 1 in, 1 out]
      n170 = Unregister For Events(event registration refnum=w27) -> ()  [unwired: 1 in, 1 out]
    }
    frame Error {
      # "Synchronize Caller Events.vi will inform Start Module.vi that the module has launched and will let the code calling Start Module.vi register for broadcasts and would permit the caller receive the broadcast that an error occurred at launch time."
      n171 = call-dynamic "Delacor_lib_QMH_Release Message Queue.vi"("error in"=w402, "Message Queue"=w395) -> ("error out"=w401:errorcluster)  [unwired: 9 in]
      n172 = call "Synchronize Caller Events.vi"("Singleton Module Admin in"=w396) -> ("error out"=w403:errorcluster)  [unwired: 9 in, 1 out]
      n173 = call "Module Name--constant.vi"() -> ("Module Name"=w399:string)  [unwired: 11 in]
      n174 = Format Into String(format string="An error occurred during initialization. %s is no longer running.", w399) -> (resulting string=w397:string)  [unwired: 2 in, 1 out]
      n175 = Merge Errors(w401, w403) -> (w404:errorcluster)
      n176 = call "Error Reported.vi"("Additional Information"=w397, "Error"=w404) -> ()  [unwired: 9 in, 1 out]
    }
  }
  n177 = Merge Errors(w18, w21) -> (w17:errorcluster)
  n178 = call "Close Module.vi"("error in"=w17, "Module Admin in"=w12) -> ("error out"=w19:errorcluster, "External Launch"=w6:bool, "Module Admin out"=w7:refnum<class "Delacor_lib_QMH_Module Admin.lvclass">)  [unwired: 7 in]
  n179 = Unregister For Events(event registration refnum=w11, error in=w19) -> (error out=w16:errorcluster)
  n180 = case "External Launch?" shown="True" w6 {
    tunnel: w16 -> [_ w405]
    frame False {
    }
    frame True {
      n181 = case shown="No Error" w405 {
        frame No Error {
          n182 = disable-structure shown="Disabled" {
            frame Disabled {
              n183 = invoke class="VI" method="FP.Close"() -> ()  [unwired: 3 in, 3 out]
            }
            frame Enabled {
            }
          }
        }
        frame Error {
          n184 = invoke class="VI" method="FP.Open"("Activate"=TRUE ("Activate?")) -> ()  [unwired: 4 in, 5 out]
        }
      }
    }
  }
  n185 = local write "Module Admin"(w7) -> ()
  n186 = Merge Errors(w16, w5, w1) -> (→"error out":errorcluster)
